vi "Run_5_of_6_Tests.vi"() -> ()   [LabVIEW 2019]
uses:
  <vilib>/Rock Robotics/WPI/ThirdParty/JAS_Junk/TrajLib/Trajectory_Library.lvlib
panel:
  out "Elliptical Region\nConstraint":bool
  out "String":string
  out "All Tests Finished":bool
  out "Diff Drive Train Sim":bool
  out "Elevator Sim":bool
  out "DARE - Ricatti":bool
  out "Discretization":bool
  # "FORMAL TRAJECTORY / CONTROL LIBRARY TEST PROCEDURE"
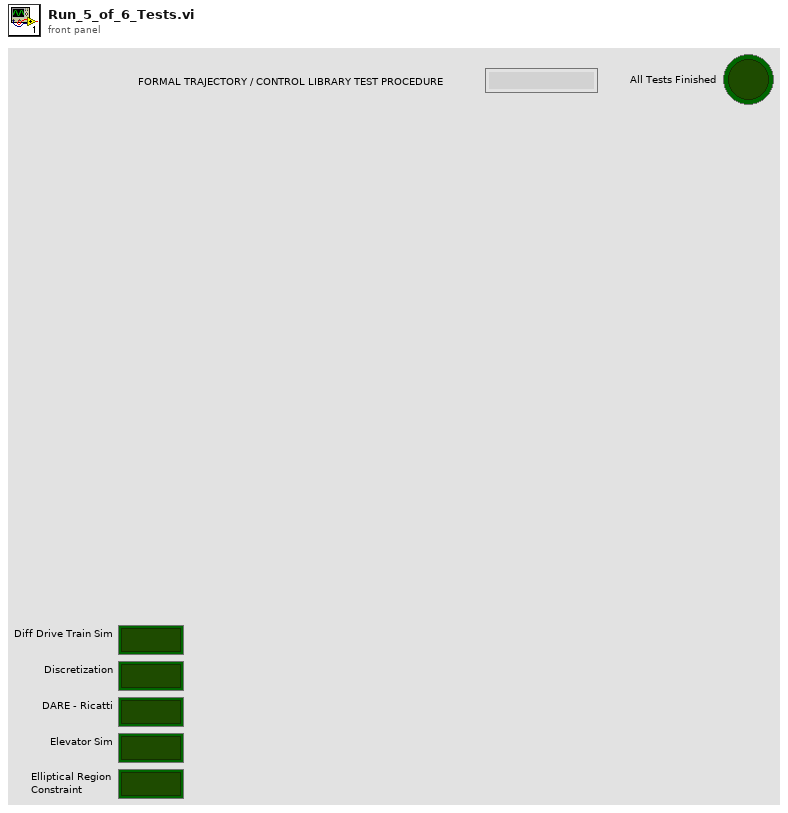
[diagram p1: front panel]
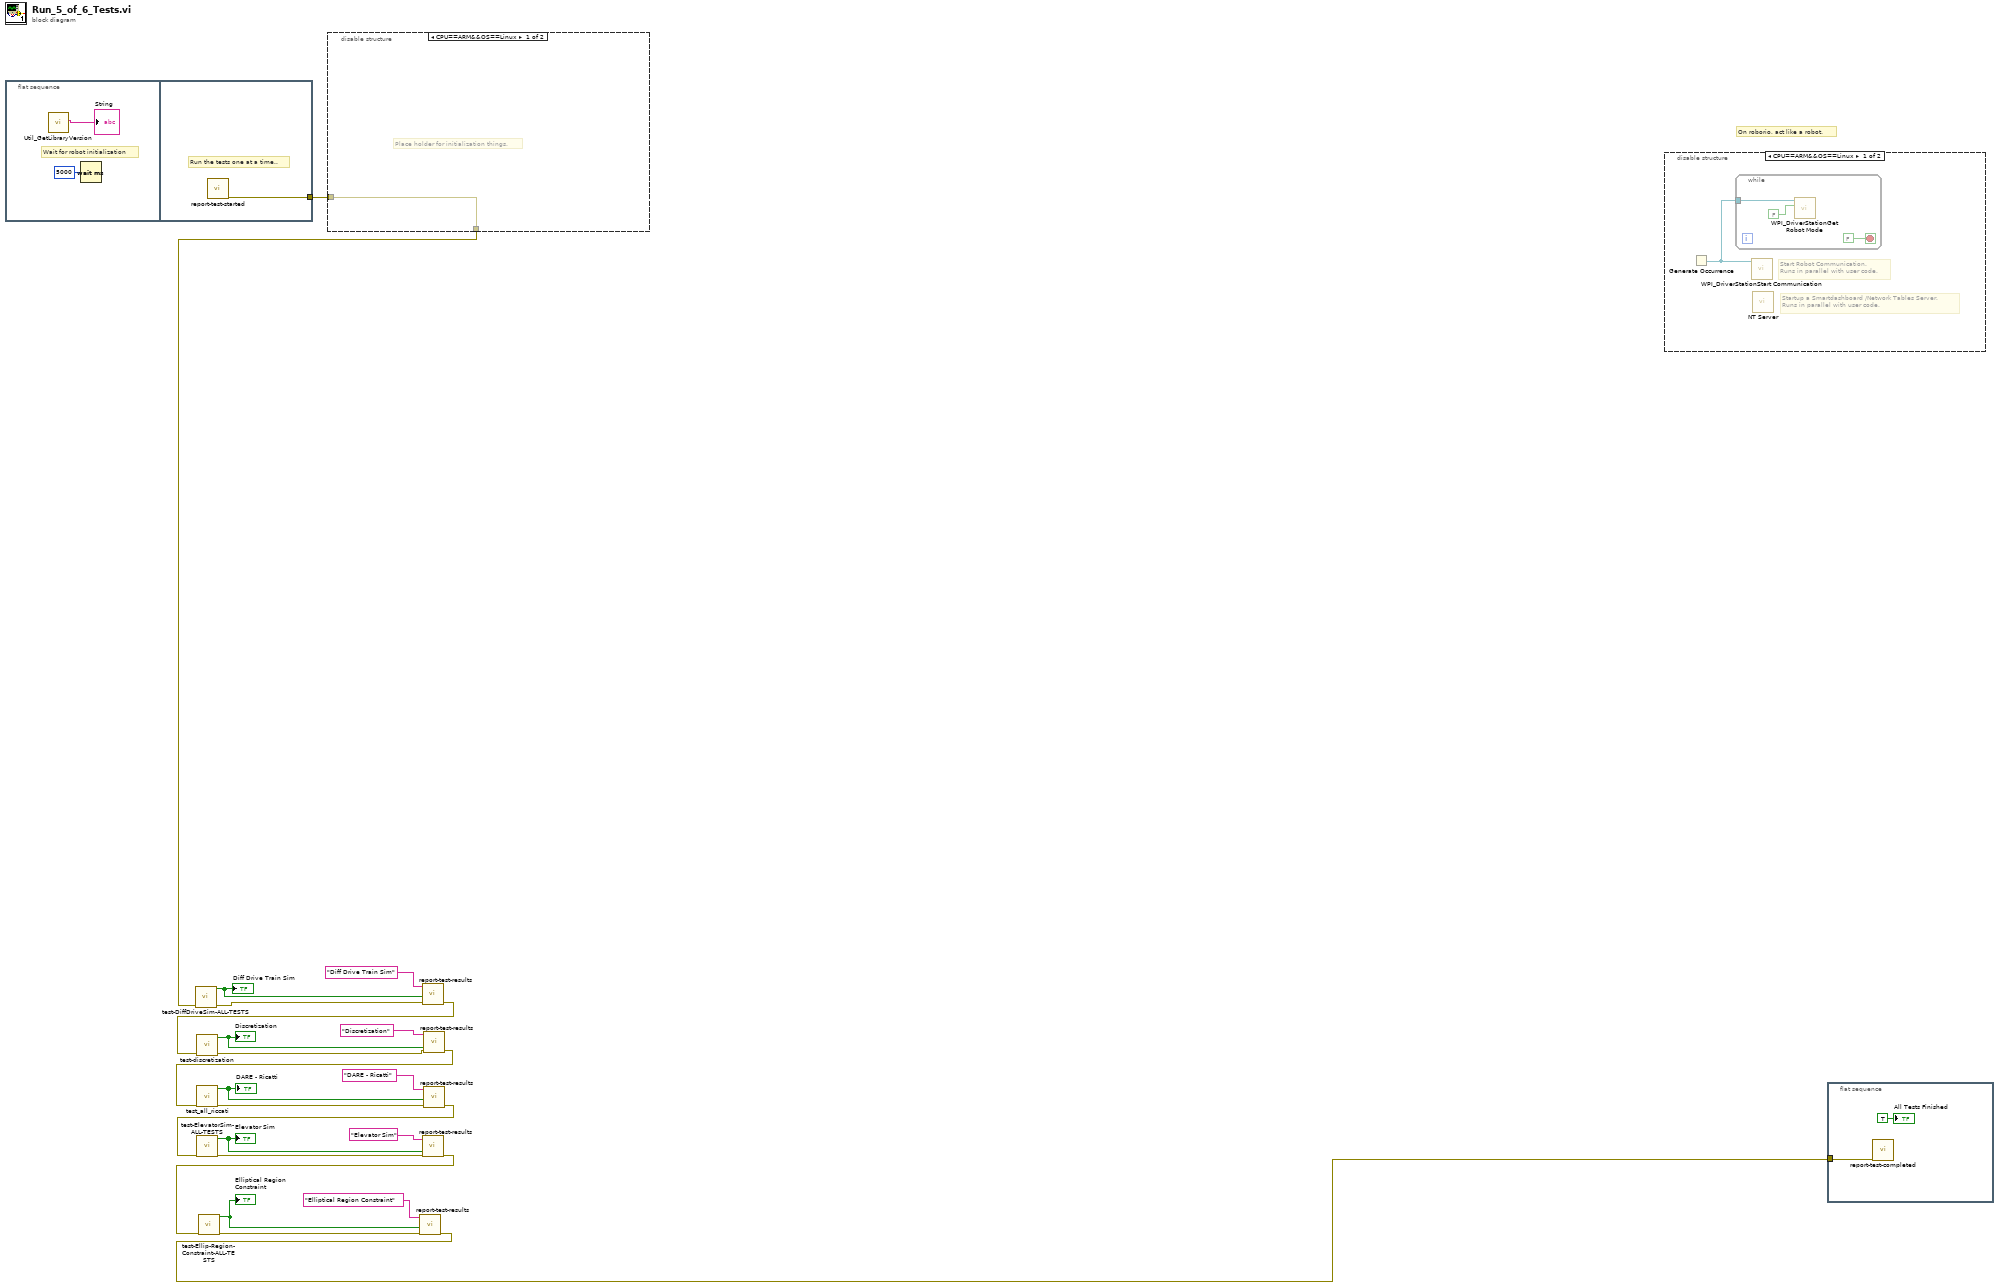
[diagram p0: block diagram]
diagram:
  # "On roborio, act like a robot."
  n1 = flat-sequence {
    tunnel: [w25] -> w7
    frame #0 {
      # "Wait for robot initialization"
      n2 = call <vilib>:"Util_GetLibraryVersion.vi"() -> ("TrajLibVersion"=→"String":string)  [unwired: 11 in]
      n3 = Wait (ms)(milliseconds to wait=u32 5000) -> ()  [unwired: 1 out]
    }
    frame #1 {
      # "Run the tests one at a time.."
      n4 = call "report-test-started.vi"() -> ("error out"=w25:errorcluster)  [unwired: 11 in]
    }
  }
  n5 = disable-structure shown="CPU==ARM&&OS==Linux" {
    disable-tunnel: w7 -> [w26 w27]
    disable-tunnel: [w26 w27] -> w6
    frame condition #0 {
      # "Place holder for initialization things."
    }
    frame condition #1 (active) {
    }
  }
  n6 = call "test-DiffDriveSim-ALL-TESTS.vi"("error in (no error)"=w6) -> ("error out"=w12:errorcluster, "All Passed"=w19:bool)  [unwired: 9 in]
  "Diff Drive Train Sim" <- w19
  n7 = call "report-test-results.vi"("error in (no error)"=w12, "TestPassed"=w19, "Test Name"="Diff Drive Train Sim") -> ("error out"=w8:errorcluster)  [unwired: 8 in]
  n8 = call "test-discretization.vi"("error in (no error)"=w8) -> ("error out"=w14:errorcluster, "All Tests Passed"=w18:bool)  [unwired: 9 in]
  "Discretization" <- w18
  n9 = call "report-test-results.vi"("error in (no error)"=w14, "TestPassed"=w18, "Test Name"="Discretization") -> ("error out"=w13:errorcluster)  [unwired: 8 in]
  n10 = call "test_all_riccati.vi"("error in (no error)"=w13) -> ("error out"=w11:errorcluster, "All Tests Passed"=w17:bool)  [unwired: 9 in]
  "DARE - Ricatti" <- w17
  n11 = call "report-test-results.vi"("error in (no error)"=w11, "TestPassed"=w17, "Test Name"="DARE - Ricatti") -> ("error out"=w9:errorcluster)  [unwired: 8 in]
  n12 = call "test-ElevatorSim-ALL-TESTS.vi"("error in (no error)"=w9) -> ("error out"=w10:errorcluster, "All Passed"=w15:bool)  [unwired: 9 in]
  "Elevator Sim" <- w15
  n13 = call "report-test-results.vi"("error in (no error)"=w10, "TestPassed"=w15, "Test Name"="Elevator Sim") -> ("error out"=w2:errorcluster)  [unwired: 8 in]
  n14 = call "test-Ellip-Region-Constraint-ALL-TESTS.vi"("error in (no error)"=w2) -> ("error out"=w4:errorcluster, "All Passed"=w3:bool)  [unwired: 9 in]
  "Elliptical Region\nConstraint" <- w3
  n15 = call "report-test-results.vi"("error in (no error)"=w4, "TestPassed"=w3, "Test Name"="Elliptical Region Constraint") -> ("error out"=w1:errorcluster)  [unwired: 8 in]
  n16 = disable-structure shown="CPU==ARM&&OS==Linux" {
    frame condition #0 {
      # "Startup a Smartdashboard /Network Tables Server.\nRuns in parallel with user code."
      # "Start Robot Communication.\nRuns in parallel with user code."
      n17 = Generate Occurrence() -> (w28:refnum<k4>)
      n18 = while {
        tunnel: w28 -> [w31]
        stop <- FALSE stop-if-true
        n19 = call <vilib>:"WPI_DriverStationGet Robot Mode.vi"("Finish"=FALSE, "DS Occurrence"=w31) -> ()  [unwired: 10 out]
      }
      n20 = call <vilib>:"WPI_DriverStationStart Communication.vi"("occurrence"=w28) -> ()  [unwired: 2 in, 9 out]
      n21 = call <vilib>:"NT Server.vi"() -> ()  [unwired: 12 in]
    }
    frame condition #1 (active) {
    }
  }
  n22 = flat-sequence {
    tunnel: w1 -> [w32]
    frame #0 {
      n23 = call "report-test-completed.vi"("error in (no error)"=w32) -> ()  [unwired: 10 in, 1 out]
      "All Tests Finished" <- TRUE ("All Tests Finished")
    }
  }
